vi "LM IRF(X)PSED and gradient v4.vi"(3 "output control":T1, 4 "data":variant, 5 "X":dbl[](array[numeric]), 6 "a":dbl[](array[numeric])) -> (0 "error out":errorcluster, 1 "f'(X,a)":dbl[][](array[numeric]), 2 "f(X,a)":dbl[](array[numeric]))   [LabVIEW 2021, in "Fits.lvlib"]
doc: "This template is the starting point for creating a model function to be passed to the Nonlinear Curve Fit.vi."
uses:
  Fits.lvlib
  <vilib>/gmath/NumericalOptimization/LM_output select.ctl
  Utilities/Utilities.lvlib
  <vilib>/gmath/NI_Gmath.lvlib
panel:
  # "Parameters:\n\nb"
  # "Data:\n\ntau, IRF order, T, {Ck, Sk, phi_k, epsilon_k}"
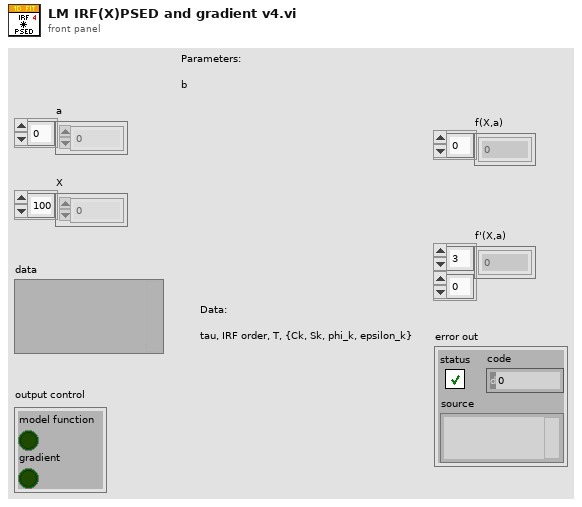
[diagram p1: front panel]
types:
  T1 = typedef "NI_Gmath.lvlib/LM_output select.ctl" = cluster{"model function":bool, "gradient":bool}
  T2 = typedef "Fits.lvlib/IRF(X)PSED Fixed Parameters v3.ctl" = cluster{"order":i32, "T":dbl, "Time Constant Array":dbl[], "{S_k, C_k, phi_k, e_k} arrays":cluster{"S_k Array":dbl[], "C_k Array":dbl[], "phi_k Array":dbl[], "e_k Array":dbl[]}, "IRF Extraction Options":T3}
  T3 = typedef "Fits.lvlib/IRF(X)PSED Extraction Options.ctl" = cluster{"Time Constant for IRF Extraction":dbl[unit], "IRF Order":i32, "Fourier Series Smoothing":T4, "Noise Threshold":dbl, "Smoothing Width":dbl, "Fourier Series Truncation":T5, "Truncation Order":i32, "Save Power Spectrum":bool, "Smoothing":bool, "Smoothing Parameter":dbl, "Smoothing Order":u32, "Method":T6}
  T4 = typedef "Fits.lvlib/Fourier Series Smoothing Option.ctl" = enum16{"None", "Lanczos Factors", "Fejer Summation"}
  T5 = typedef "Fits.lvlib/Fourier Series Truncation.ctl" = enum16{"Automatic", "Fixed"}
  T6 = typedef "Fits.lvlib/IRF Extraction Method.ctl" = enum16{"Direct", "Topless", "Toeplitz"}
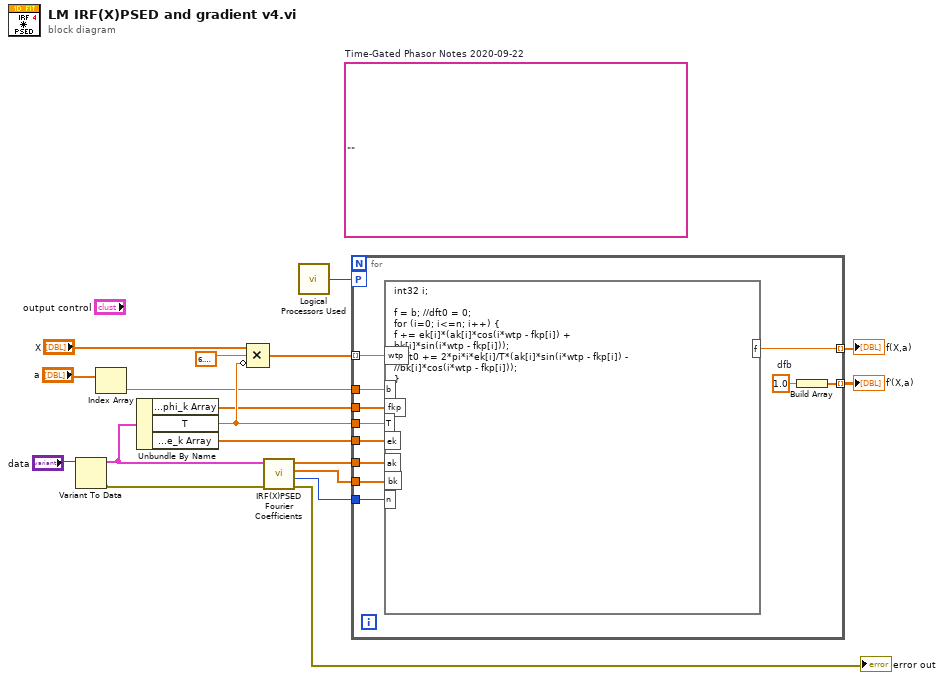
[diagram p0: block diagram]
diagram:
  (unwired) ""  # Time-Gated Phasor Notes 2020-09-22
  n1 = Variant To Data(Variant="data") -> (data=w7:T2, error out=w4:errorcluster)  [unwired: 2 in]
  n2 = Index Array(array="a") -> (element=w10:dbl)  [unwired: 1 in]
  n3 = Unbundle By Name(w7) -> ("{S_k, C_k, phi_k, e_k} arrays.phi_k Array"=w9:dbl[], "T"=w11:dbl, "{S_k, C_k, phi_k, e_k} arrays.e_k Array"=w8:dbl[])
  n4 = Compound Arithmetic op=MULTIPLY("X", 6.283185307179586, invert w11) -> (w12:dbl[])
  n5 = call "IRF(X)PSED Fourier Coefficients.vi"("Error In"=w4, "IRF*PSED fixed Parameters"=w7) -> ("Error Out"=→"error out":errorcluster, "Optimal Order"=w2:i32, "[b_k]"=w5:dbl[], "[a_k]"=w6:dbl[])  [unwired: 4 in, 2 out]
  n6 = call "Logical Processors Used.vi"() -> ("# Logical Processor Used"=w1:i32)  [unwired: 6 in]
  n7 = for {
    tunnel: w12 -> [w29] mode=indexing
    tunnel: [w28] -> w18 mode=indexing
    tunnel: [w27] -> w15 mode=indexing
    tunnel: w10 -> [w26]
    tunnel: w2 -> [w25]
    tunnel: w6 -> [w22]
    tunnel: w5 -> [w21]
    tunnel: w9 -> [w23]
    tunnel: w11 -> [w20]
    tunnel: w8 -> [w19]
    workers-P: w1 -> [_]
    w24 = 1.0  # dfb
    n8 = formula code="int32 i;\n\nf = b; //dft0 = 0;\nfor (i=0; i<=n; i++) {\nf += ek[i]*(ak[i]*cos(i*wtp - fkp[i]) +\nbk[i]*sin(i*wtp - fkp[i]));\n//dft0 += 2*pi*i*ek[i]/T*(ak[i]*sin(i*wtp - fkp[i]) -\n//bk[i]*cos(i*wtp - fkp[i]));\n}"("wtp"=w29, "b"=w26, "n"=w25, "fkp"=w23, "ak"=w22, "bk"=w21, "T"=w20, "ek"=w19) -> ("f"=w28:dbl)
    n9 = Build Array(w24) -> (w27:dbl[])
  }
  "f(X,a)" <- w18
  "f'(X,a)" <- w15
